vi "QNET_Rotpen_Construct_State_Sim.vi"(2 "alpha (rad)":dbl, 3 "theta (rad)":dbl, 4 "theta_r (rad)":dbl) -> (0 "x cluster":T1, 1 "x array":dbl[](array[numeric]))   [LabVIEW 2010]
uses:
  <vilib>/Simulation/Implementation/Shared/SIMSCR Execution Mode.ctl
  <vilib>/Simulation/Scripting/Companion Diagram/SimConfigNode/SimDog.xnode
  <vilib>/Simulation/Scripting/Companion Diagram/SimConfigNode/SimParams.ctl
  <vilib>/Simulation/Scripting/Companion Diagram/SimConfigNode/_simSolvers.ctl
  <vilib>/Simulation/Implementation/XNodeFramework/SimXNode/SimX.xnode
  <vilib>/Simulation/Shared/_Datatypes/SIM SISO Transfer Function.ctl
  <vilib>/Simulation/ContinuousLinear/Implementation/NILVSim Transfer Function Direct.llb/SIM Transfer Function Direct (SISO).vi
  <vilib>/Simulation/Implementation/Shared/NILVSim_Manager.vi
  <vilib>/Simulation/Implementation/Shared/NILVSim_GetModelError.vi
  <vilib>/Simulation/Implementation/Shared/NILVSim_FinalizeModel.vi
  <vilib>/Simulation/Implementation/Shared/NILVSim_GetSimErrorInfo.vi
  <vilib>/Simulation/Implementation/Shared/NILVSim_GenerateString.vi
  <vilib>/Simulation/Implementation/Shared/NILVSim_GetBlockNameAndCallChain.vi
  <vilib>/Simulation/Implementation/Shared/NILVSim_GetSimErrorString.vi
  <vilib>/Simulation/Implementation/Shared/NILVSim_GetBlockNameAndCallChainSizes.vi
  <vilib>/Simulation/Implementation/Shared/NILVSim_GetBlockNameAndCallChain Core.vi
  <vilib>/Simulation/Implementation/Shared/SIM Unbundle Sim Info.vi
  <vilib>/Simulation/Implementation/Shared/SIM SimErrorHandler.vi
  <vilib>/Simulation/Implementation/Shared/SIM Bundle Sim Info.vi
  <vilib>/Simulation/Implementation/Shared/NILVSim_Initialize.vi
  <vilib>/dlg_ctls.llb/Space Constant.vi
  <vilib>/Simulation/Implementation/Shared/NI_SIM_Implementation.lvlib
panel:
  in  "x":T1
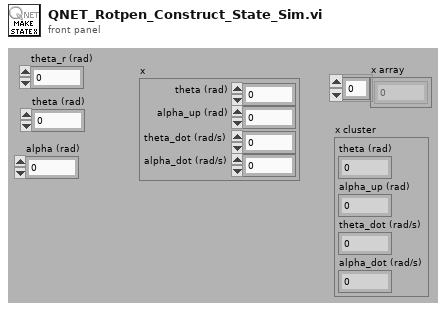
[diagram p1: front panel]
types:
  T1 = cluster{"theta (rad)":dbl, "alpha_up (rad)":dbl, "theta_dot (rad/s)":dbl, "alpha_dot (rad/s)":dbl}
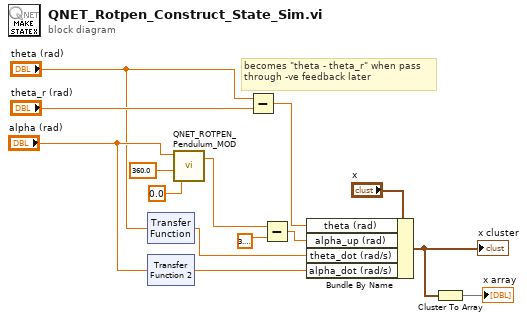
[diagram p0: block diagram]
diagram:
  # "becomes \"theta - theta_r\" when pass through -ve feedback later"
  n1 = xnode ("Transfer Function")("input u(k)"="theta (rad)") -> ("output y(k)"=w6:dbl)  [unwired: 2 in, 1 out]
  n2 = xnode ("Transfer Function 2")("input u(k)"="alpha (rad)") -> ("output y(k)"=w7:dbl)  [unwired: 2 in, 1 out]
  n3 = call "QNET_ROTPEN_Pendulum_MOD.vi"("offset (deg)"=0.0, "mod angle (deg)"=360.0, "gamma (rad)"="alpha (rad)") -> ("gamma mod (rad)"=w11:dbl)  [unwired: 1 in, 1 out]
  n4 = Subtract(x="theta (rad)", y="theta_r (rad)") -> (x-y=w1:dbl)
  n5 = Subtract(x=w11, y=3.141592653589793) -> (x-y=w14:dbl)
  n6 = Bundle By Name(cluster="x", "theta (rad)"=w1, "alpha_up (rad)"=w14, "theta_dot (rad/s)"=w6, "alpha_dot (rad/s)"=w7) -> (w4:T1)
  "x cluster" <- w4
  n7 = Cluster To Array(cluster=w4) -> (array=→"x array":dbl[])
